vi "WinCondNumTests.vi"() -> ()   [LabVIEW 2020]
panel:
  out "Test results":cluster{"Success?":bool, "data in":i32[]}[](array[cluster])
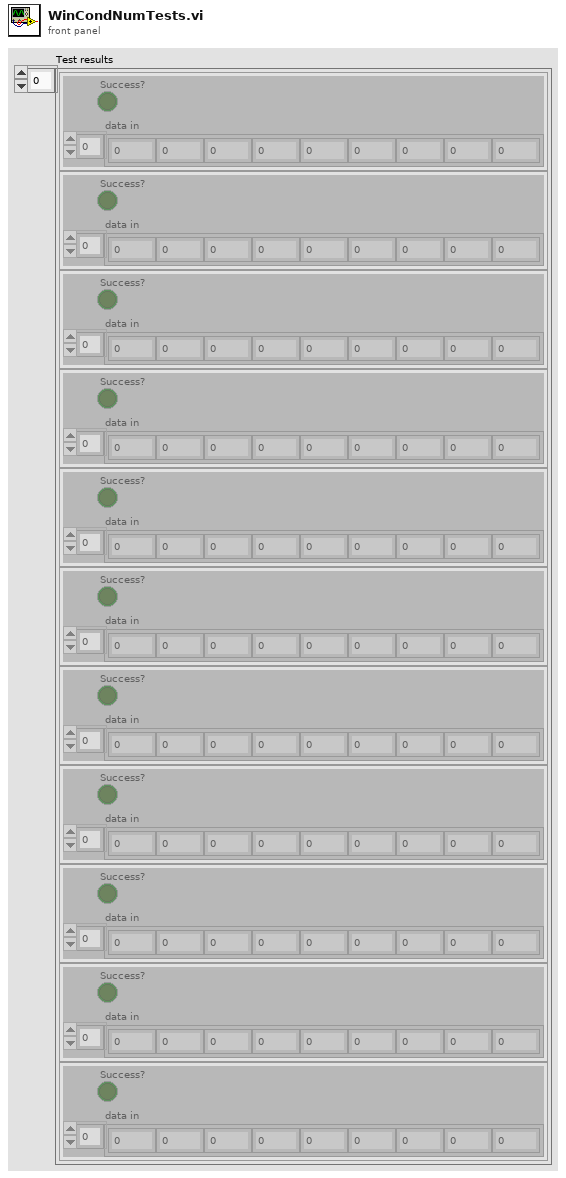
[diagram p1: front panel]
types:
  T1 = cluster{"data in":i32[], "test end":bool, "test ind":i32[]}
  T2 = cluster{"data in":i32[], "test end":bool, "test ind":i32[]}[]
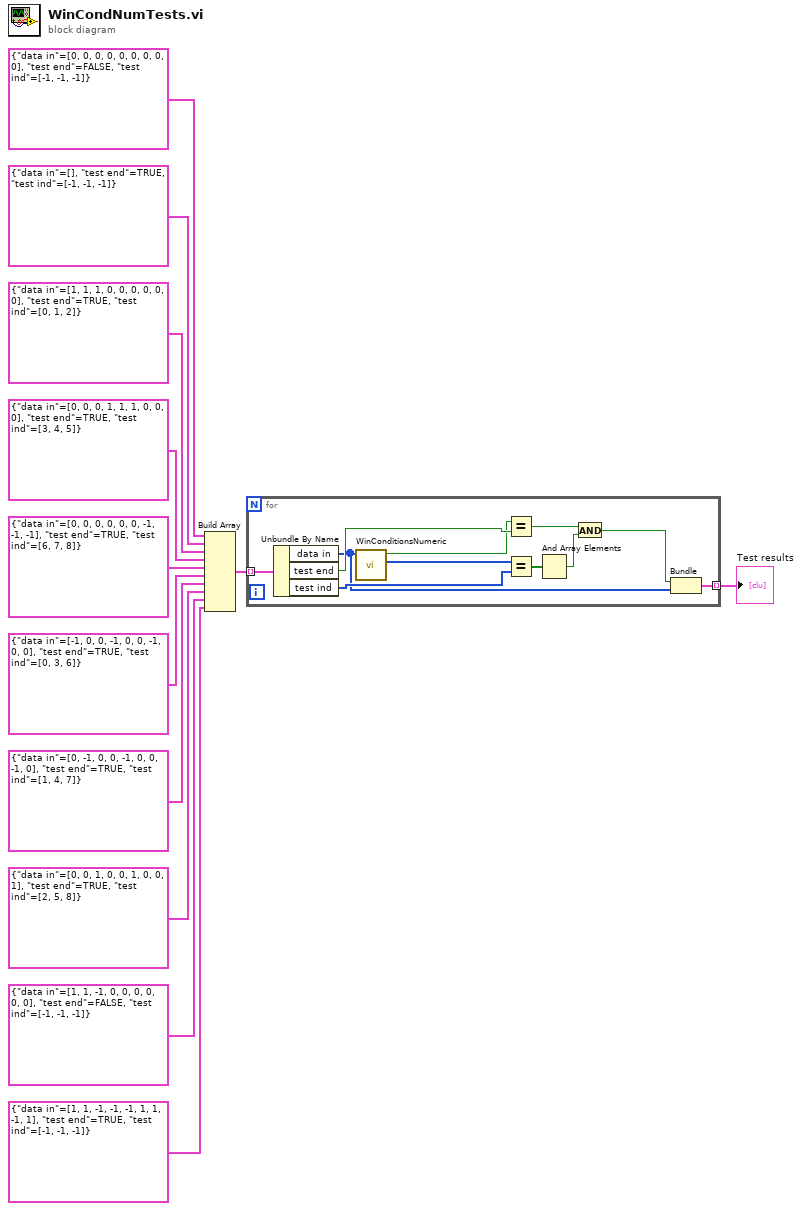
[diagram p0: block diagram]
diagram:
  n1 = Build Array(T1 {"data in"=[0, 0, 0, 0, 0, 0, 0, 0, 0], "test end"=FALSE, "test ind"=[-1, -1, -1]}, T1 {"data in"=[], "test end"=TRUE, "test ind"=[-1, -1, -1]}, T1 {"data in"=[1, 1, 1, 0, 0, 0, 0, 0, 0], "test end"=TRUE, "test ind"=[0, 1, 2]}, T1 {"data in"=[0, 0, 0, 1, 1, 1, 0, 0, 0], "test end"=TRUE, "test ind"=[3, 4, 5]}, T1 {"data in"=[0, 0, 0, 0, 0, 0, -1, -1, -1], "test end"=TRUE, "test ind"=[6, 7, 8]}, T1 {"data in"=[-1, 0, 0, -1, 0, 0, -1, 0, 0], "test end"=TRUE, "test ind"=[0, 3, 6]}, T1 {"data in"=[0, -1, 0, 0, -1, 0, 0, -1, 0], "test end"=TRUE, "test ind"=[1, 4, 7]}, T1 {"data in"=[0, 0, 1, 0, 0, 1, 0, 0, 1], "test end"=TRUE, "test ind"=[2, 5, 8]}, T1 {"data in"=[1, 1, -1, 0, 0, 0, 0, 0, 0], "test end"=FALSE, "test ind"=[-1, -1, -1]}, T1 {"data in"=[1, 1, -1, -1, -1, 1, 1, -1, 1], "test end"=TRUE, "test ind"=[-1, -1, -1]}) -> (w2:T2)
  n2 = for {
    tunnel: w2 -> [w23] mode=indexing
    tunnel: [w14] -> w1 mode=indexing
    n3 = Unbundle By Name(w23) -> ("data in"=w15:i32[], "test end"=w22:bool, "test ind"=w20:i32[])
    n4 = call "WinConditionsNumeric.vi"("NumericGameboard"=w15) -> ("LineIndices"=w19:i8[], "End?"=w21:bool)  [unwired: 9 in]
    n5 = Equal?(x=w21, y=w22) -> (x = y?=w18:bool)
    n6 = Equal?(x=w19, y=w20) -> (x = y?=w17:bool[])
    n7 = And Array Elements(Boolean array=w17) -> (logical AND=w13:bool)
    n8 = And(x=w18, y=w13) -> (x .and. y?=w16:bool)
    n9 = Bundle(w16, "data in"=w15) -> (w14:cluster{bool, "data in":i32[]})  [unwired: 1 in]
  }
  "Test results" <- w1
